vi "SDF Small Gasifier RT - Process Logic.vi"() -> ()   [LabVIEW 2013]
uses:
  SDF Small Gasifier RT - Process Logic States.ctl
  <vilib>/NI/Current Value Table/DataTypes/String_Write.vi
  <vilib>/NI/Current Value Table/DataTypes/Boolean_Write.vi
  <vilib>/NI/Current Value Table/Static Read.vi
  <vilib>/NI/Current Value Table/DataTypes/Boolean_Static Read.vi
  <vilib>/NI/AMC/Read Termination Message.vi
  <vilib>/NI/Current Value Table/Type to Enum.vi
  <vilib>/NI/Current Value Table/DataTypes/String_Type To Enum.vi
  <vilib>/NI/Current Value Table/DataTypes/Boolean_Type To Enum.vi
  <vilib>/NI/AMC/Create Single Message.vi
  <vilib>/NI/Current Value Table/FGVs/CVT Globals.vi
  <vilib>/NI/Current Value Table/FGVs/Tag Memory.vi
  <vilib>/NI/Current Value Table/Memory Block.vi
  <vilib>/NI/Current Value Table/DataTypes/Boolean_Memory Block.vi
  <vilib>/NI/AMC/Globals.vi
  <vilib>/NI/Current Value Table/DataTypes/String_Memory Block.vi
  <vilib>/NI/Current Value Table/Current Value Table.lvlib
  <vilib>/NI/AMC/AMC.lvlib
panel:
  out "Value 2":string
  out "s? t:f":T1
  out "Message Name":string
  in  "Process States":T1
  in  "Stop":bool
  out "Index":i32
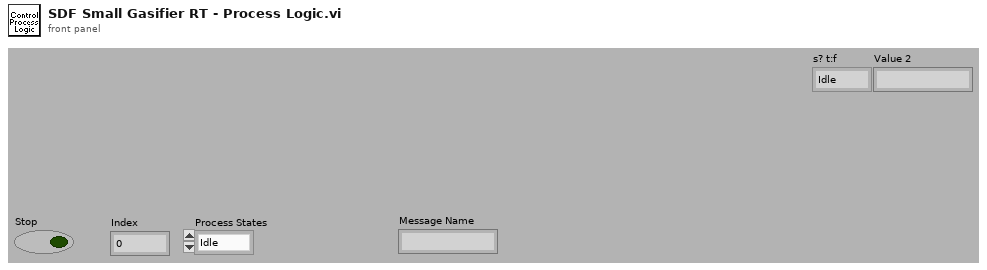
[diagram p1: front panel]
types:
  T1 = typedef "SDF Small Gasifier RT - Process Logic States.ctl" = enum16{"Idle", "Start", "Fill", "Heat", "Cook", "Drain", "Finish"}
  T2 = typedef "AMC.lvlib/Message Queue.ctl" = refnum<queue>
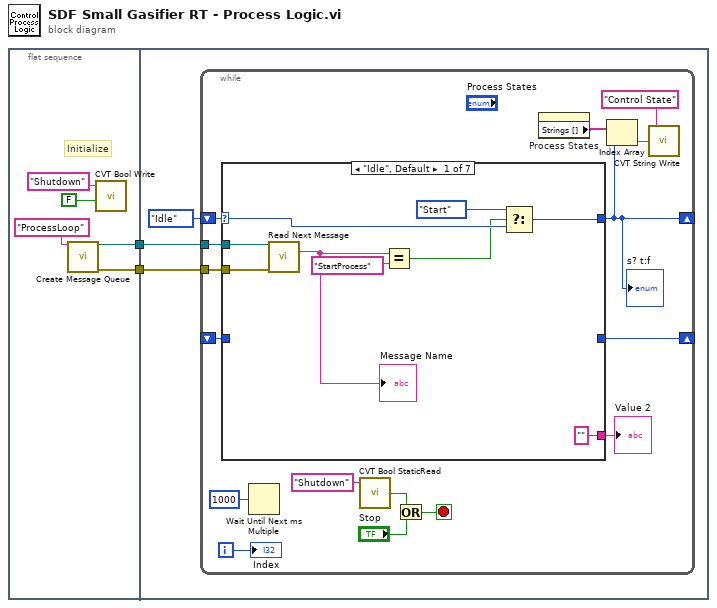
[diagram p0: block diagram]
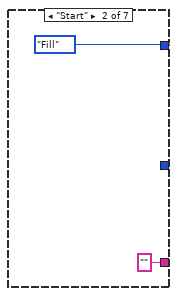
[diagram p2: hidden frame]
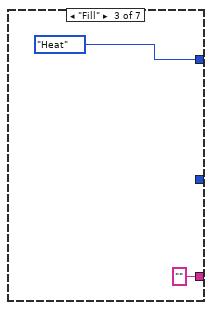
[diagram p3: hidden frame]
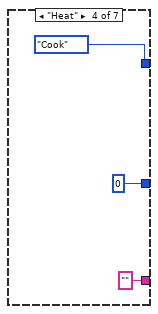
[diagram p4: hidden frame]
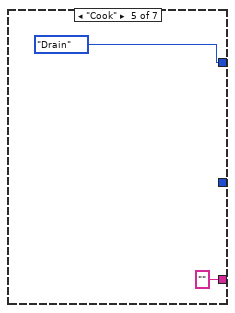
[diagram p5: hidden frame]
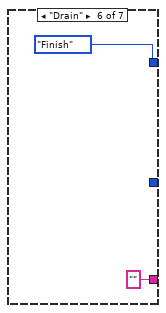
[diagram p6: hidden frame]
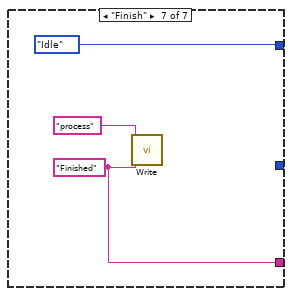
[diagram p7: hidden frame]
diagram:
  n1 = flat-sequence {
    tunnel: [w5] -> w2
    tunnel: [w3] -> w1
    tunnel: w2 -> [w9]
    tunnel: w1 -> [w8]
    frame #0 {
      # "Initialize"
      n2 = call <vilib>:"Create Message Queue.vi"("message queue name"="ProcessLoop" ("Message Queue Name")) -> ("message queue out"=w5:T2, "error out"=w3:errorcluster)  [unwired: 13 in]
      n3 = call <vilib>:"CVT Bool Write.vi"("Value"=FALSE, "Tag Name"="Shutdown") -> ()  [unwired: 3 in, 1 out]
    }
    frame #1 {
      n4 = while {
        shift-right: [w12] -> _
        shift-left: SDF_Small_Gasifier_RT_-_Process_Logic_States."Idle" ("Process States") -> [w26]
        shift-right: [w24] -> _
        shift-left: _ -> [w25]
        tunnel: w9 -> [w14]
        tunnel: w8 -> [w13]
        i -> [w23]
        stop <- w19 stop-if-true
        n5 = case shown="\"Idle\", Default" w26 {
          selector: w26 -> [w35 _ _ _ _ _ _]
          tunnel: [w31 SDF_Small_Gasifier_RT_-_Process_Logic_States."Fill" ("Process States") SDF_Small_Gasifier_RT_-_Process_Logic_States."Heat" ("t") SDF_Small_Gasifier_RT_-_Process_Logic_States."Cook" ("t") SDF_Small_Gasifier_RT_-_Process_Logic_States."Drain" ("t") SDF_Small_Gasifier_RT_-_Process_Logic_States."Finish" ("t") SDF_Small_Gasifier_RT_-_Process_Logic_States."Idle" ("t")] -> w12
          tunnel: [_ _ _ 0 _ _ _] -> w24
          tunnel: w25 -> [_ _ _ _ _ _ _]
          tunnel: w14 -> [w29 _ _ _ _ _ _]
          tunnel: w13 -> [w28 _ _ _ _ _ _]
          tunnel: ["" ("Value") "" ("Value") "" ("Value") "" ("Value") "" ("Value") "" ("Value") w47] -> w11
          frame "Idle", Default {
            n6 = call <vilib>:"Read Next Message.vi"("message queue in"=w29, "error in"=w28) -> ("message name"=w27:string)  [unwired: 6 in, 7 out]
            "Message Name" <- w27
            n7 = Equal?(x=w27, y="StartProcess" ("Tag Name")) -> (x = y?=w32:bool)
            n8 = Select(t=SDF_Small_Gasifier_RT_-_Process_Logic_States."Start", s=w32, f=w35) -> (s? t:f=w31:T1)
          }
          frame "Start" {
          }
          frame "Fill" {
          }
          frame "Heat" {
          }
          frame "Cook" {
          }
          frame "Drain" {
          }
          frame "Finish" {
            w47 = "Finished" ("Value")
            n9 = call-poly <vilib>:"Write.vi"("Value"=w47, "Tag Name"="process") -> ()  [unwired: 9 in, 1 out]
          }
        }
        "s? t:f" <- w12
        "Value 2" <- w11
        n10 = Wait Until Next ms Multiple(millisecond multiple=u32 1000) -> ()  [unwired: 1 out]
        n11 = call <vilib>:"CVT Bool StaticRead.vi"("Tag Name"="Shutdown") -> ("Value"=w20:bool)  [unwired: 3 in, 1 out]
        n12 = Or(x=w20, y="Stop") -> (x .or. y?=w19:bool)
        n13 = property on="Process States" class="Enum (strict)"() -> ("Strings []"=w17:string[])  [unwired: 2 in, 2 out]
        n14 = Index Array(array=w17, index=w12) -> (element=w16:string)
        n15 = call <vilib>:"CVT String Write.vi"("Value"=w16, "Tag Name"="Control State") -> ()  [unwired: 3 in, 1 out]
        "Index" <- w23
      }
    }
  }
